vi "lockin - Set REF phase equals zero.vi"(8 "error in (no error)":errorcluster, 9 "Reset Phase":bool, 11 "Instrument.DAQ":refnum<class "Instrument.DAQ.lvclass">) -> (0 "error out":errorcluster, 3 "Instrument.DAQ out":refnum<class "Instrument.DAQ.lvclass">)   [LabVIEW 2019, in "Instrument.Lockin.lvlib" / "Instrument.DAQ.lvclass"]
uses:
  Instrument.DAQ.lvclass
  Instrument.DAQ.lvclass/Instrument.DAQ.ctl
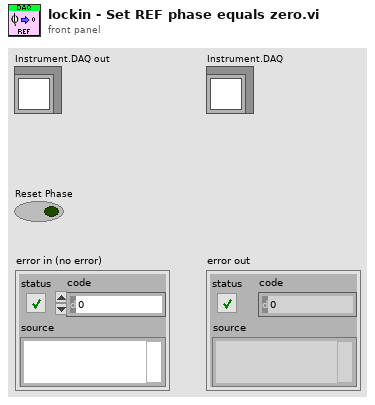
[diagram p1: front panel]
types:
  T1 = typedef "Instrument.Lockin.lvlib/Instrument.DAQ.lvclass/REF.Channel--Cluster--Array.ctl" = T2[]
  T2 = typedef "Instrument.Lockin.lvlib/Instrument.DAQ.lvclass/REF.Channel--Cluster.ctl" = cluster{"Enable?":bool, "Channel":i32, "Frequency":dbl, "Phase":dbl, "TC":dbl, "Roll-Off":i32}
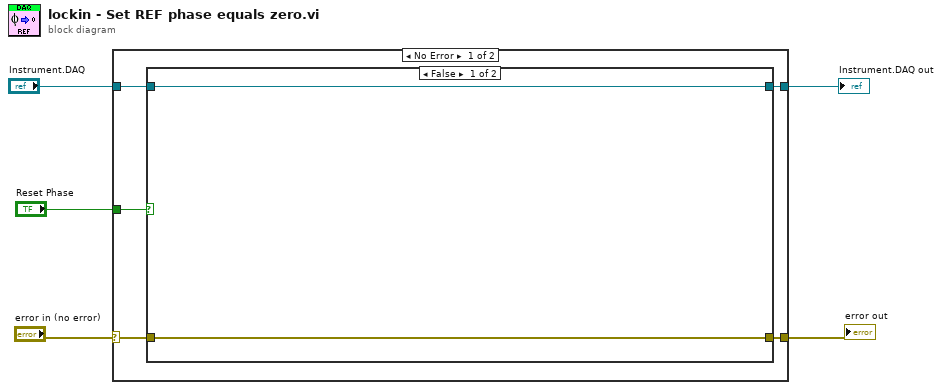
[diagram p0: block diagram]
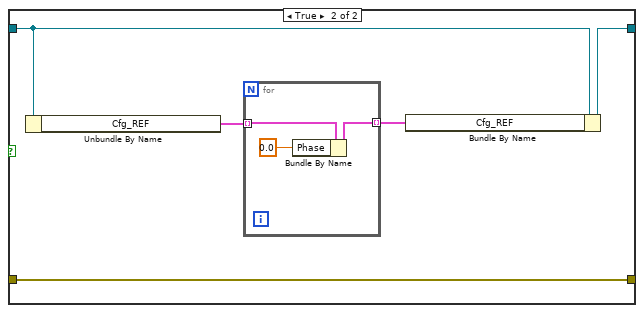
[diagram p2: hidden frame]
diagram:
  n1 = case shown="No Error" "error in (no error)" {
    selector: "error in (no error)" -> [w7 w22]
    tunnel: "Instrument.DAQ" -> [w10 w21]
    tunnel: [w9 w21] -> w4
    tunnel: [w6 w22] -> w2
    tunnel: "Reset Phase" -> [w8 _]
    frame No Error {
      n2 = case shown="False" w8 {
        tunnel: w10 -> [w12 w16]
        tunnel: [w12 w15] -> w9
        tunnel: w7 -> [w11 w13]
        tunnel: [w11 w13] -> w6
        frame False {
        }
        frame True {
          n3 = Unbundle By Name(w16) -> ("Cfg_REF"=w17:T1)
          n4 = for {
            tunnel: w17 -> [w20] mode=indexing
            tunnel: [w18] -> w14 mode=indexing
            n5 = Bundle By Name(cluster=w20, "Phase"=0.0) -> (w18:T2)
          }
          n6 = Bundle By Name(cluster=w16, "Cfg_REF"=w14) -> (w15:refnum<class "Instrument.DAQ.lvclass">)
        }
      }
    }
    frame Error {
    }
  }
  "Instrument.DAQ out" <- w4
  "error out" <- w2
